vi "Do.vi"(8 "error in (no error)":errorcluster, 10 "Actor in":refnum<class "Actor.lvclass">, 11 "test Msg":refnum<class "test Msg.lvclass">) -> (0 "error out":errorcluster, 2 "Actor out":refnum<class "Actor.lvclass">)   [LabVIEW 2024, in "Active.lvlib" / "test Msg.lvclass"]
doc: "This VI delivers the message to the actor by calling the appropriate method(s) on the actor."
uses:
  test Msg.lvclass
  test Msg.lvclass/test Msg.ctl
  eb60ab54-563e-4109-9ce4-a3c53cd9b356.vi
  Active/Active.lvclass
  C:/Users/uspoaotto/OneDrive - Oregon Tool/Desktop/working copies/stateMachineActor/src/Nested State Machine Actors/Automation Controller/Automation Controller/Automation Controller.lvclass
  C:/Users/uspoaotto/OneDrive - Oregon Tool/Desktop/working copies/stateMachineActor/src/State Pattern Actor/State Machine/State Machine/State Machine.lvclass
  C:/Program Files (x86)/National Instruments/LabVIEW 2024/vi.lib/ActorFramework/Actor/Actor.lvclass
  C:/Users/uspoaotto/OneDrive - Oregon Tool/Desktop/working copies/stateMachineActor/src/Nested State Machine Actors/Event Messages/Event Messages/Event Messages.lvclass
  C:/Users/uspoaotto/OneDrive - Oregon Tool/Desktop/working copies/stateMachineActor/src/Nested State Machine Actors/Active/Active/Active.lvclass
  <vilib>/ActorFramework/Actor/Actor.lvclass
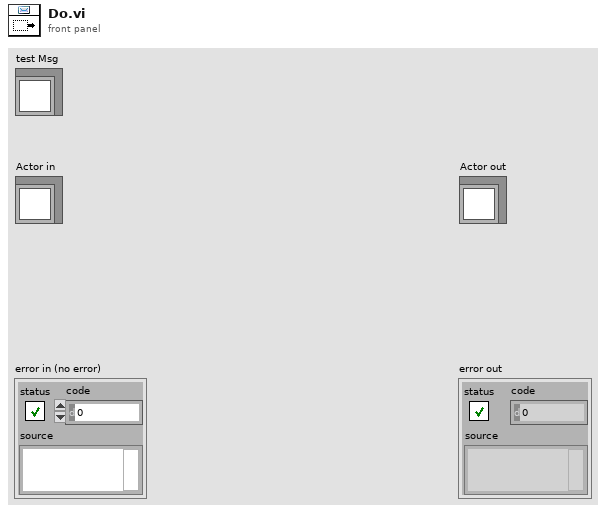
[diagram p1: front panel]
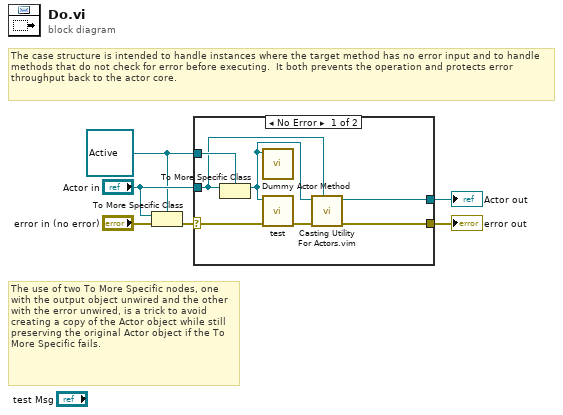
[diagram p0: block diagram]
diagram:
  w2 = refnum<class "Active.lvclass"> refnum ("Actor in")
  # "The use of two To More Specific nodes, one with the output object unwired and the other with the error unwired, is a trick to avoid creating a copy of the Actor object while still preserving the original Actor object if the To More Specific fails."
  # "The case structure is intended to handle instances where the target method has no error input and to handle methods that do not check for error before executing.  It both prevents the operation and protects error throughput back to the actor core."
  n1 = To More Specific Class(target class=w2, reference="Actor in", error in="error in (no error)") -> (error out=w1:errorcluster)  [unwired: 1 out]
  n2 = case shown="No Error" w1 {
    selector: w1 -> [w13 w15]
    tunnel: [w8 w15] -> w6
    tunnel: [w9 w14] -> w5
    tunnel: "Actor in" -> [w10 w14]
    tunnel: w2 -> [w11 _]
    frame No Error {
      n3 = To More Specific Class(target class=w11, reference=w10) -> (specific class reference=w12:refnum<class "Active.lvclass">)  [unwired: 1 in, 1 out]
      n4 = call <resource>:"Dummy Actor Method.vi"("Actor in"=w12) -> ()  [unwired: 9 in, 2 out]
      n5 = call-dynamic "test.vi"("error in (no error)"=w13, "Active in"=w12) -> ("error out"=w7:errorcluster)  [unwired: 8 in, 1 out]
      n6 = call "Casting Utility For Actors.vim"("type"=w10, "error in (no error)"=w7, "Actor in"=w12) -> ("error out"=w8:errorcluster, "Actor out"=w9:refnum<class "Actor.lvclass">)  [unwired: 7 in]
    }
    frame Error {
      # "If type check fails, pass the original object out again."
    }
  }
  "error out" <- w6
  "Actor out" <- w5
